vi "Day 02 Part 2.vi"(11 "Input":string) -> (3 "Output":dbl)   [LabVIEW 2021]
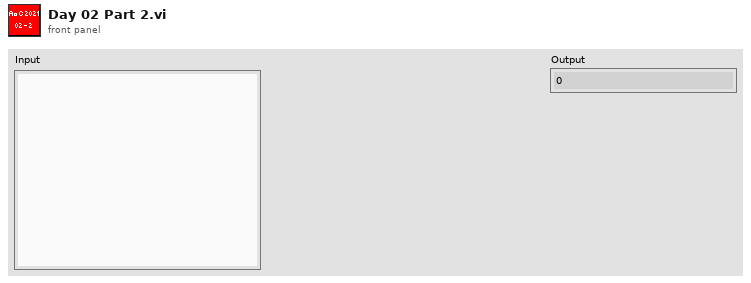
[diagram p1: front panel]
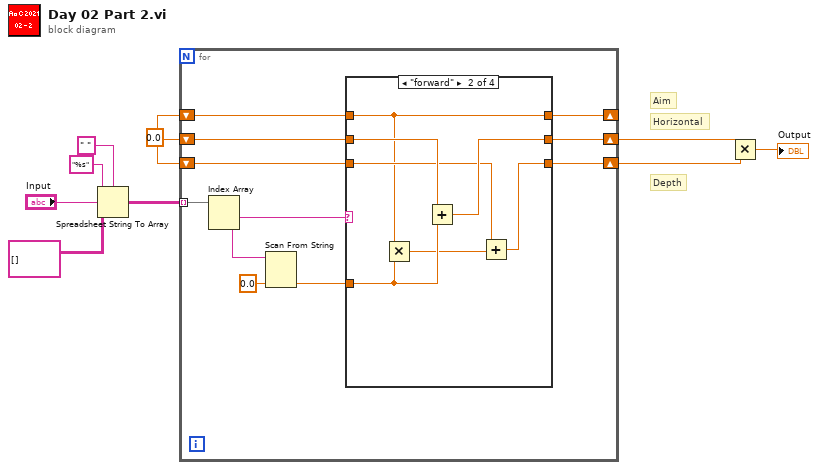
[diagram p0: block diagram]
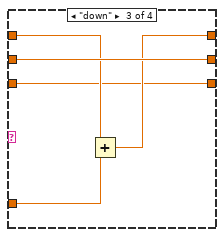
[diagram p3: hidden frame]
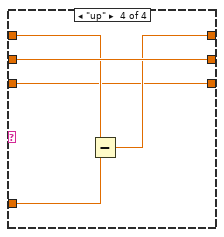
[diagram p4: hidden frame]
diagram:
  w1 = 0.0
  # "Depth"
  # "Horizontal"
  # "Aim"
  n1 = Spreadsheet String To Array(delimiter (Tab)=" ", format string="%s", spreadsheet string="Input", array type (2D Dbl)=string[][] []) -> (array=w5:string[][])
  n2 = for {
    tunnel: w5 -> [w20] mode=indexing
    shift-right: [w17] -> w3
    shift-left: w1 -> [w16]
    shift-right: [w12] -> w4
    shift-left: w1 -> [w18]
    shift-right: [w10] -> _
    shift-left: w1 -> [w11]
    n3 = Index Array(array=w20) -> (element #1=w19:string, element #2=w15:string)  [unwired: 2 in]
    n4 = Scan From String(input string=w15, default 1=0.0 ("default value 1")) -> (output 1=w14:dbl)  [unwired: 3 in, 3 out]
    n5 = case shown="\"forward\"" w19 {
      tunnel: w18 -> [w22 w30 w35 w40]
      tunnel: [w23 w26 w31 w36] -> w17
      tunnel: w16 -> [w23 w25 w31 w36]
      tunnel: w14 -> [_ w28 w34 w39]
      tunnel: [w22 w29 w35 w40] -> w12
      tunnel: w11 -> [w21 w24 w33 w38]
      tunnel: [w21 w24 w32 w37] -> w10
      frame Default {
      }
      frame "forward" {
        n6 = Multiply(x=w24, y=w28) -> (x*y=w27:dbl)
        n7 = Add(x=w30, y=w28) -> (x+y=w29:dbl)
        n8 = Add(x=w25, y=w27) -> (x+y=w26:dbl)
      }
      frame "down" {
        n9 = Add(x=w33, y=w34) -> (x+y=w32:dbl)
      }
      frame "up" {
        n10 = Subtract(x=w38, y=w39) -> (x-y=w37:dbl)
      }
    }
  }
  n11 = Multiply(x=w4, y=w3) -> (x*y=→"Output":dbl)
